vi "CSM - Post Message(SimMode).vi"(8 "Error In (no error)":errorcluster, 9 "Target Module":string="A", 10 "Arguments (\"\")":string, 11 "State":string="DoA") -> (0 "error out":errorcluster)   [LabVIEW 2014, in "Communicable State Machine.lvlib"]
doc: "Post a message to CSM specified.\n\n<b>Inputs:</b>\n - <b>Target Module</b>:Target CSM Module name.\n - <b>State</b>: Message to post.\n - <b>Arguments (\"\")</b>: Argument of the message.\n - <b>Error In (no error)</b>: Error cluster\n\n<b>Outputs:</b>\n - <b>error out</b>: Error cluster"
uses:
  Communicable State Machine.lvlib
  CSM - Message Type.ctl
  _Support/Priority Queue/Priority Queue.lvclass/Priority Queue.ctl
  _Support/Process/CSMP-Async Call.vi
  _Support/GlobalEvent/GEvt-Generate Status Log.vi
  _Support/Process/CSMP-Broadcast.vi
  _Support/GlobalEvent/GEvt-Generate Interrupt Log.vi
  _Support/GlobalEvent/GEvt-Generate Register Log.vi
  _Support/Process/CSMP-Register Status.vi
  _Support/GlobalEvent/GEvt-Generate Unregister Log.vi
  _Support/Process/CSMP-Unregister Status.vi
  _Support/Process/CSMP-Sync Call.vi
  _Support/CSMQ/_CSMObj-Unlock.vi
  _Support/Process/CSMP-PostPostMsg.vi
  _Support/Process/CSMP-PostSendMsg.vi
  _Support/CSMQ/_CSMObj-Lock State.vi
  _Support/Common/Splite Reason String Part.vi
  _Support/Common/Trim Single line Text.vi
  CSM - Convert Argument to Error.vi
  _Support/CSMQ/_CSMOFGV Release.vi
  _Support/Common/Remove Comments from Line.vi
  _Support/Common/Splite Single-line Message.vi
  _Support/Common/Parse Next Single-line State.vi
  _Support/CSMQ/_CSMOFGV Dequeue.vi
  CSM - Convert Error to Argument.vi
  _Support/CSMQ/_CSMObj-Log Error if in a Remote Session.vi
  _Support/GlobalEvent/GEvt-Generate State Change Log.vi
  _Support/GlobalEvent/GEvt-Generate Remaining States Log.vi
  _Support/GlobalEvent/GEvt-Generate Module Destroyed Log.vi
  _Support/GlobalEvent/GEvt-Generate Complete Log.vi
  _Support/GlobalEvent/GEvt-Generate Module Created Log.vi
  _Support/CSMQ/_CSMObj-Message Check.vi
  _Support/CSMQ/_CSMObj-Enqueue Cross-Module Message.vi
  _Support/CSMQ/_CSMOFGV Get.vi
  _Support/FGV-BroadcastRegistry/Cache-Broadcast Registry Search Result.vi
  CSM - Register Status Change.vi
  CSM - Unregister Status Change.vi
  _Support/Common/Hex Str to U8 Data.vi
  CSM - Revert Arguments-Safe String.vi
  <vilib>/addons/_JKI Toolkits/State Machine/_JKI_lib_State_Machine.llb/Add State(s) to Queue__JKI_lib_State_Machine.vi
  Utility/Build Internal State String.vi
  _Support/Common/Concatenate State with Arguments.vi
  _Support/Common/U8 Data to Hex Str.vi
  <vilib>/addons/_JKI Toolkits/State Machine/_JKI_lib_State_Machine.llb/Build State String with Arguments__JKI_lib_State_Machine.vi
  _Support/Priority Queue/Dequeue Element.vi
  CSM - Make String Arguments Safe.vi
  _Support/Priority Queue/Enqueue Element.vi
  CSM - Keywords.vi
  _Support/CSMQ/_CSMOFGV.vi
  _Support/FGV-BroadcastRegistry/FGV-BroadcastRegistry.vi
  _Support/FGV-BroadcastRegistry/global-Broadcast Cache Change Flag.vi
  _Support/GlobalEvent/FGV-StatusChangeEventRef.vi
  _Support/CSMQ/_CSMOFGV Obtain.vi
  _Support/GlobalEvent/FGV-GlobalEventRef.vi
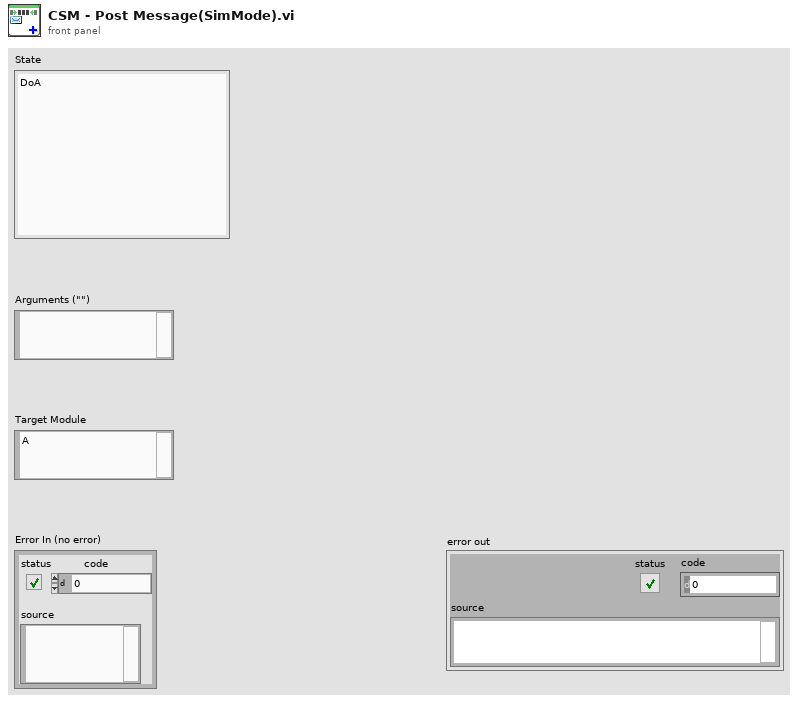
[diagram p1: front panel]
types:
  T1 = typedef "Communicable State Machine.lvlib/CSM - Message Type.ctl" = enum16{"Async", "Async without Reply", "Sync"}
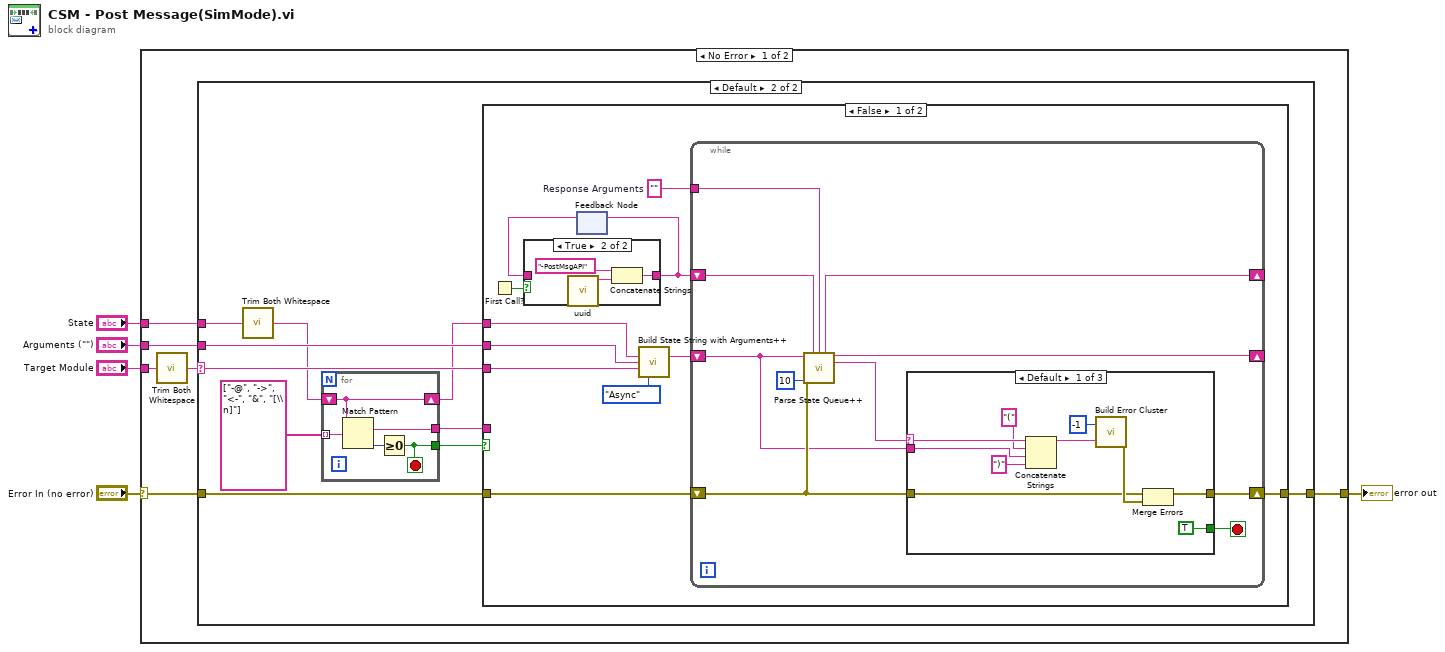
[diagram p0: block diagram]
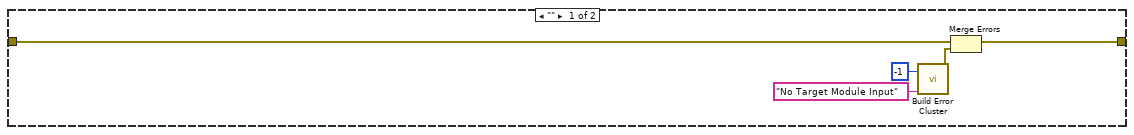
[diagram p2: hidden frame]
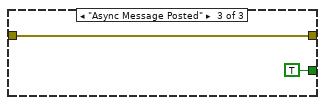
[diagram p5: hidden frame]
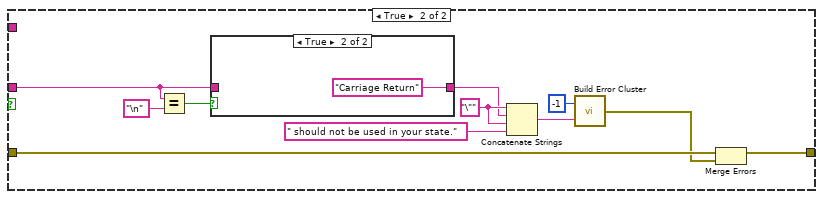
[diagram p6: hidden frame]
diagram:
  n1 = case shown="No Error" "Error In (no error)" {
    selector: "Error In (no error)" -> [w9 w83]
    tunnel: "State" -> [w6 _]
    tunnel: [w10 w83] -> w3
    tunnel: "Arguments (\"\")" -> [w7 _]
    tunnel: "Target Module" -> [w11 _]
    frame No Error {
      n2 = call "Trim Both Whitespace.vi"("string"=w11) -> ("trimmed string"=w8:string)  [unwired: 1 in]
      n3 = case shown="Default" w8 {
        selector: w8 -> [_ w25]
        tunnel: w6 -> [_ w21]
        tunnel: w7 -> [_ w26]
        tunnel: [w15 w24] -> w10
        tunnel: w9 -> [w16 w23]
        frame "" {
          n4 = call "Build Error Cluster.vi"("String to Prepend to source (\"\")"="No Target Module Input" ("String to Prepend to source (\"\")"), "code"=-1) -> ("error out"=w14:errorcluster)
          n5 = Merge Errors(w16, w14) -> (w15:errorcluster)
        }
        frame Default {
          n6 = call "Trim Both Whitespace.vi"("string"=w21) -> ("trimmed string"=w17:string)  [unwired: 1 in]
          n7 = for {
            shift-right: [w82] -> w20
            shift-left: w17 -> [w82]
            tunnel: string[] ["-@", "->", "<-", "&", "[\\n]"] -> [w81] mode=indexing
            tunnel: [w79] -> w18
            tunnel: [w78] -> w19
            stop <- w78 stop-if-true
            n8 = Match Pattern(string=w82, regular expression=w81) -> (match substring=w79:string, offset past match=w80:i32)  [unwired: 1 in, 2 out]
            n9 = Greater Or Equal To 0?(x=w80) -> (x >= 0?=w78:bool)
          }
          n10 = case shown="False" w19 {
            tunnel: w26 -> [w37 _]
            tunnel: w25 -> [w36 _]
            tunnel: [w34 w67] -> w24
            tunnel: w23 -> [w33 w68]
            tunnel: w20 -> [w28 _]
            tunnel: w18 -> [_ w65]
            frame False {
              w35 = ""  # Response Arguments
              n11 = First Call?() -> (First Call?: T/F=w31:bool)
              n12 = feedback #1() -> (w30:string)  [unwired: 1 in]
              n13 = case shown="True" w31 {
                tunnel: [w38 w39] -> w29
                tunnel: w30 -> [w38 _]
                frame False {
                }
                frame True {
                  n14 = call "uuid.vi"() -> ("UUID"=w40:string)  [unwired: 11 in]
                  n15 = Concatenate Strings("-PostMsgAPI" ("Name(\"\" to use uuid)"), w40) -> (w39:string)
                }
              }
              n16 = feedback-in #1(w29) -> ()
              n17 = call "Build State String with Arguments++.vi"("State"=w28, "Arguments (\"\")"=w37, "Target Module (\"\")"=w36, "Type"=CSM_-_Message_Type."Async") -> ("State with Arguments"=w32:string)  [unwired: 11 in]
              n18 = while {
                tunnel: w35 -> [w50]
                shift-right: [w48] -> w34
                shift-left: w33 -> [w47]
                shift-right: [w44] -> _
                shift-left: w32 -> [w45]
                shift-right: [w43] -> _
                shift-left: w29 -> [w46]
                stop <- w42 stop-if-true
                n19 = call "Parse State Queue++.vi"("State Queue"=w45, "Name(\"\" to use uuid)"=w46, "Response Arguments"=w50, "Error In (no error)"=w47, "Response Timeout(5000ms)"=10 ("Response Timeout(1000ms)")) -> ("Name Used"=w43:string, "Remaining States"=w44:string, "Current State"=w49:string)  [unwired: 5 in, 3 out]
                n20 = case shown="Default" w49 {
                  selector: w49 -> [w60 _ _]
                  tunnel: [w57 w62 w64] -> w48
                  tunnel: w47 -> [w56 w62 w64]
                  tunnel: w45 -> [w55 _ _]
                  tunnel: [TRUE _ TRUE] -> w42
                  frame Default {
                    n21 = Concatenate Strings(w60, "(" ("string"), w55, ")" ("string")) -> (w59:string)
                    n22 = call "Build Error Cluster.vi"("String to Prepend to source (\"\")"=w59, "code"=-1) -> ("error out"=w58:errorcluster)
                    n23 = Merge Errors(w56, w58) -> (w57:errorcluster)
                  }
                  frame "Async Response" {
                  }
                  frame "Async Message Posted" {
                  }
                }
              }
            }
            frame True {
              w72 = "\"" ("string")
              n24 = Equal?(x=w65, y="\n" ("regular expression")) -> (x = y?=w69:bool)
              n25 = case shown="True" w69 {
                tunnel: [w76 "Carriage Return" ("State")] -> w71
                tunnel: w65 -> [w76 _]
                frame False {
                }
                frame True {
                }
              }
              n26 = Concatenate Strings(w72, w71, w72, " should not be used in your state." ("String to Prepend to source (\"\")")) -> (w73:string)
              n27 = call "Build Error Cluster.vi"("String to Prepend to source (\"\")"=w73, "code"=-1) -> ("error out"=w66:errorcluster)
              n28 = Merge Errors(w68, w66) -> (w67:errorcluster)
            }
          }
        }
      }
    }
    frame Error {
    }
  }
  "error out" <- w3
